vi "Run Process.vi"(8 "error in (no error)":errorcluster, 9 "Processes":cluster{"VI":refnum<vi>, "Parameters":variant}[](array[cluster]), 11 "Async in":refnum<class "VS Inline Async API.lvclass">) -> (0 "error out":errorcluster, 3 "Async out":refnum<class "VS Inline Async API.lvclass">)   [LabVIEW 2023, in "VS Inline Async API.lvlib" / "VS Inline Async API.lvclass"]
uses:
  VS Inline Async API.lvclass
  VS Inline Async API.lvclass/VS Inline Async API.ctl
  Process/Process.lvclass
  Process/Process.lvclass/Process.ctl
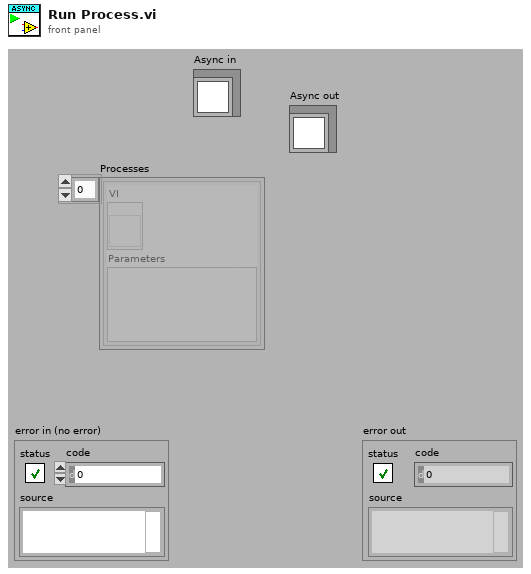
[diagram p1: front panel]
types:
  T1 = cluster{"read mode":enum16{"polling", "blocking"}, "write mode":enum16{"polling", "blocking"}}
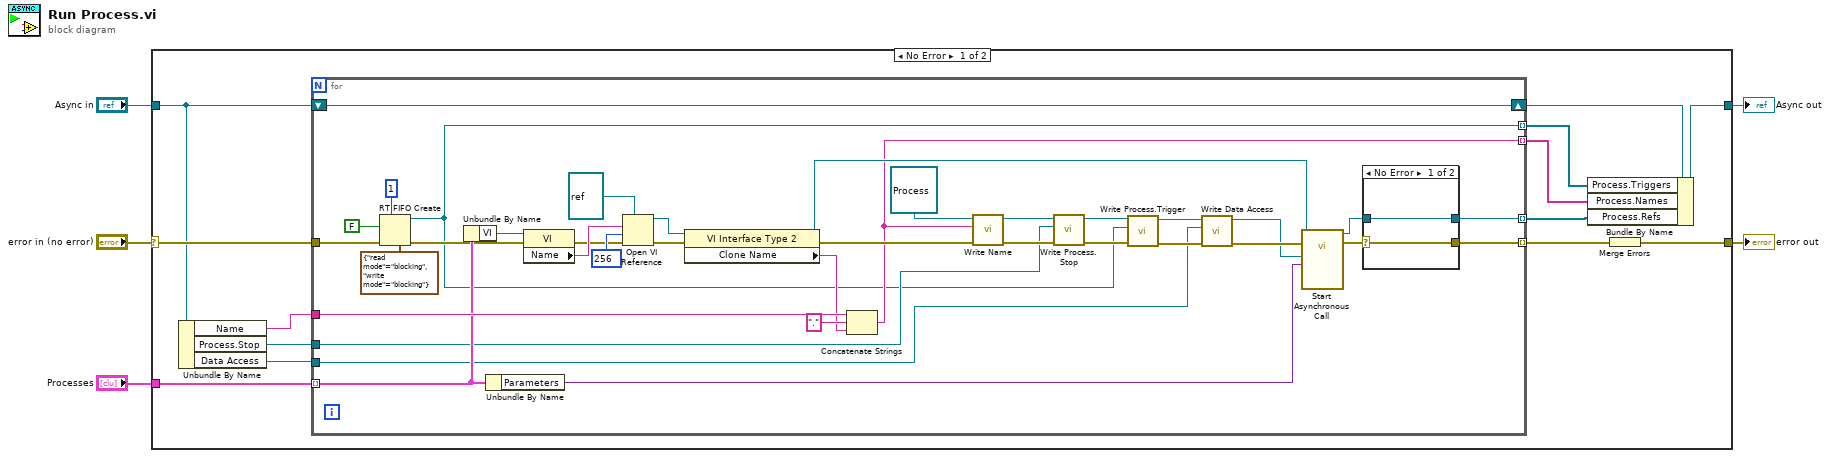
[diagram p0: block diagram]
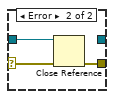
[diagram p2: hidden frame]
diagram:
  n1 = case shown="No Error" "error in (no error)" {
    selector: "error in (no error)" -> [w17 w62]
    tunnel: [w15 w62] -> w5
    tunnel: "Processes" -> [w16 _]
    tunnel: "Async in" -> [w11 w61]
    tunnel: [w12 w61] -> w1
    frame No Error {
      n2 = Unbundle By Name(w11) -> ("Name"=w10:string, "Process.Stop"=w9:refnum<data-value>, "Data Access"=w7:refnum<class "Data Access Engine.lvclass">)
      n3 = for {
        tunnel: [w55] -> w18 mode=indexing
        tunnel: [w54] -> w14 mode=indexing
        tunnel: w17 -> [w37]
        tunnel: w16 -> [w45] mode=indexing
        shift-right: [w50] -> w13
        shift-left: w11 -> [w50]
        tunnel: w10 -> [w49]
        tunnel: w9 -> [w21]
        tunnel: [w22] -> w8 mode=indexing
        tunnel: w7 -> [w19]
        tunnel: [w20] -> w6 mode=indexing
        n4 = RT FIFO Create(1:FALSE, 3:w37, 4:u32 1 ("size (10)"), 7:T1 {"read mode"=enum."blocking", "write mode"=enum."blocking"} ("r/w modes (polling,polling)")) -> (8:w20:refnum<k33>, 11:w36:errorcluster)  [unwired: 4 in, 1 out]
        n5 = Unbundle By Name(w45) -> ("VI"=w46:refnum<vi>)
        n6 = Unbundle By Name(w45) -> ("Parameters"=w44:variant)
        n7 = property class="VI"(reference=w46, error in=w36) -> (error out=w40:errorcluster, "Name"=w48:string)  [unwired: 1 out]
        n8 = Open VI Reference(type specifier VI Refnum (for type only)=refnum<vi> refnum, vi path=w48, options=256, error in (no error)=w40) -> (vi reference=w42:refnum<vi>, error out=w43:errorcluster)  [unwired: 2 out]
        n9 = property class="VI Interface Type 2"(reference=w42, error in=w43) -> (reference out=w41:refnum<vi>, error out=w26:errorcluster, "Clone Name"=w39:string)
        n10 = Concatenate Strings(w49, "." ("string"), w39) -> (w22:string)
        n11 = call "Write Name.vi"("error in (no error)"=w26, "Name"=w22, "Process in"=refnum<class "Process.lvclass"> refnum ("VS Inline Async API.lvlib:Process.lvclass")) -> ("error out"=w28:errorcluster, "Process out"=w30:refnum<class "Process.lvclass">)  [unwired: 7 in]
        n12 = call "Write Process.Stop.vi"("error in (no error)"=w28, "Process.Stop"=w21, "Process in"=w30) -> ("error out"=w32:errorcluster, "Process out"=w31:refnum<class "Process.lvclass">)  [unwired: 7 in]
        n13 = call "Write Process.Trigger.vi"("error in (no error)"=w32, "Process.Trigger"=w20, "Process in"=w31) -> ("error out"=w27:errorcluster, "Process out"=w29:refnum<class "Process.lvclass">)  [unwired: 7 in]
        n14 = call "Write Data Access.vi"("error in (no error)"=w27, "Data Access"=w19, "Process in"=w29) -> ("error out"=w25:errorcluster, "Process out"=w24:refnum<class "Process.lvclass">)  [unwired: 7 in]
        n15 = call-by-ref "Start Asynchronous Call"(reference=w41, error in=w25, "Parameters"=w44, "Process"=w24) -> (reference out=w52:refnum<vi>, error out=w53:errorcluster)  [unwired: 10 in]
        n16 = case shown="No Error" w53 {
          selector: w53 -> [w57 w60]
          tunnel: w52 -> [w56 w59]
          tunnel: [w57 w58] -> w55
          tunnel: [w56 _] -> w54
          frame No Error {
          }
          frame Error {
            n17 = Close Reference(reference=w59, error in (no error)=w60) -> (error out=w58:errorcluster)
          }
        }
      }
      n18 = Bundle By Name(cluster=w13, "Process.Triggers"=w6, "Process.Names"=w8, "Process.Refs"=w14) -> (w12:refnum<class "VS Inline Async API.lvclass">)
      n19 = Merge Errors(w18) -> (w15:errorcluster)
    }
    frame Error {
    }
  }
  "error out" <- w5
  "Async out" <- w1
